vi "RealTimeStiffness.vi"() -> ()   [LabVIEW 2017]
uses:
  <vilib>/Utility/file.llb/Read Delimited Spreadsheet (DBL).vi
  <vilib>/Analysis/NI_AALBase.lvlib
panel:
  in  "Size":i32=500
  out "XY Graph":cluster{dbl[], dbl[]}[](graph)
  in  "Size":i32=60
  out "Histogram Graph":T1(graph)
  in  "stop":bool
  out "all rows":dbl[][](array[numeric])
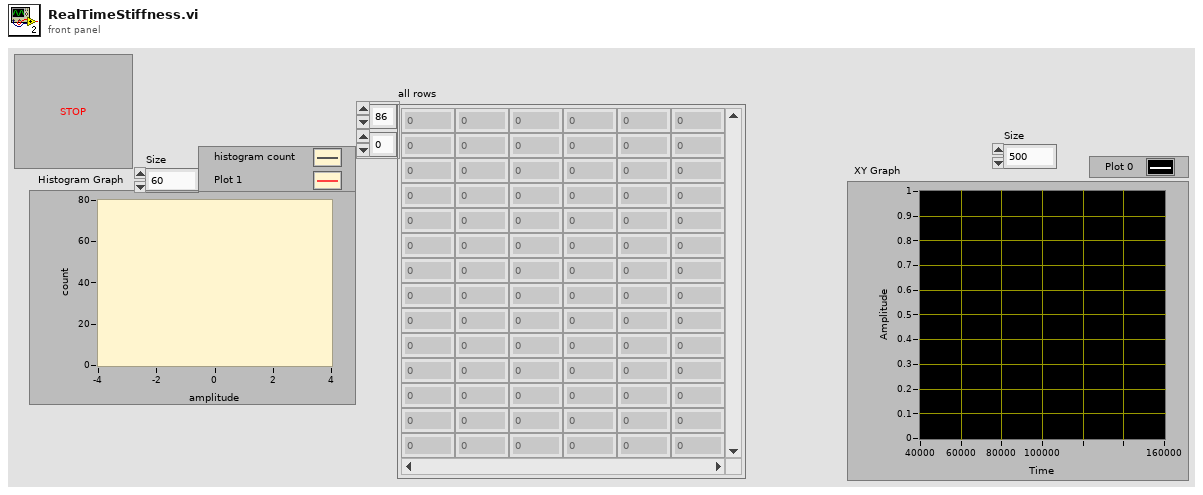
[diagram p1: front panel]
types:
  T1 = cluster{"X Values":dbl[], "Histogram: h(x)":i32[]}[]
  T2 = cluster{"X Values":dbl[], "Histogram: h(x)":i32[]}
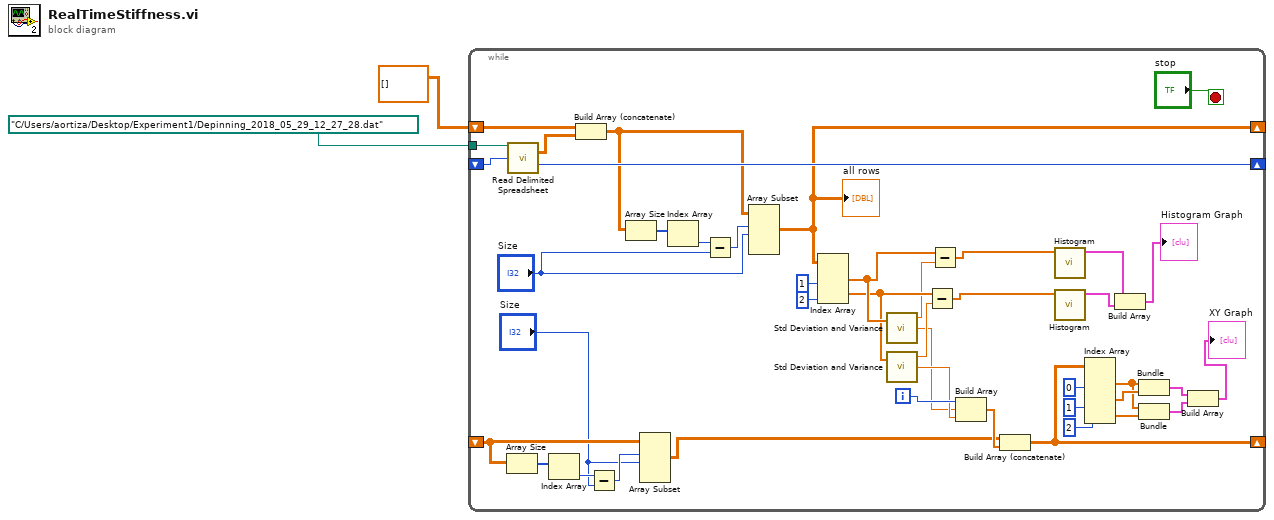
[diagram p0: block diagram]
diagram:
  n1 = while {
    tunnel: path "C:/Users/aortiza/Desktop/Experiment1/Depinning_2018_05_29_12_27_28.dat" ("file path (dialog if empty)") -> [w45]
    shift-right: [w35] -> _
    shift-left: dbl[][] [] -> [w38]
    shift-right: [w41] -> _
    shift-left: _ -> [w40]
    shift-right: [w16] -> _
    shift-left: _ -> [w20]
    i -> [w25]
    stop <- "stop" stop-if-true
    n2 = Array Size(array=w20) -> (size(s)=w22:i32[])
    n3 = call-poly <vilib>:"Read Delimited Spreadsheet.vi"("file path (dialog if empty)"=w45, "start of read offset (chars.:0)"=w40) -> ("all rows"=w37:dbl[][], "mark after read (chars.)"=w41:i32)  [unwired: 8 in, 4 out]
    n4 = Index Array(array=w22) -> (element=w19:i32)  [unwired: 1 in]
    n5 = Build Array (concatenate)(w38, w37) -> (w36:dbl[][])
    n6 = Subtract(x=w19, y="Size") -> (x-y=w18:i32)
    n7 = Array Size(array=w36) -> (size(s)=w44:i32[])
    n8 = Array Subset(array=w20, index (row)=w18, length (row)="Size") -> (w17:dbl[][])  [unwired: 2 in]
    n9 = Index Array(array=w44) -> (element=w43:i32)  [unwired: 1 in]
    n10 = Subtract(x=w43, y="Size") -> (x-y=w42:i32)
    n11 = Array Subset(array=w36, index (row)=w42, length (row)="Size") -> (w35:dbl[][])  [unwired: 2 in]
    "all rows" <- w35
    n12 = Index Array(array=w35, index (col) #1=1 ("disabled index (col)"), index (col) #2=2 ("index (col)")) -> (element #1=w28:dbl[], element #2=w27:dbl[])  [unwired: 2 in]
    n13 = call <vilib>:"Std Deviation and Variance.vi"("X"=w28) -> ("mean"=w24:dbl, "standard deviation"=w4:dbl)  [unwired: 1 in, 1 out]
    n14 = call <vilib>:"Std Deviation and Variance.vi"("X"=w27) -> ("mean"=w6:dbl, "standard deviation"=w5:dbl)  [unwired: 1 in, 1 out]
    n15 = Subtract(x=w27, y=w6) -> (x-y=w26:dbl[])
    n16 = Subtract(x=w28, y=w24) -> (x-y=w29:dbl[])
    n17 = Build Array(w25, w4, w5) -> (w23:dbl[])
    n18 = Build Array (concatenate)(w17, w23) -> (w16:dbl[][])
    n19 = call <vilib>:"Histogram.vi"("X"=w29) -> ("Histogram Graph"=w31:T2)  [unwired: 7 in, 3 out]
    n20 = call <vilib>:"Histogram.vi"("X"=w26) -> ("Histogram Graph"=w32:T2)  [unwired: 7 in, 3 out]
    n21 = Index Array(array=w16, index (col) #1=0 ("disabled index (col)"), index (col) #2=1 ("index (col)"), index (col) #3=2 ("index (col)")) -> (element #1=w11:dbl[], element #2=w12:dbl[], element #3=w10:dbl[])  [unwired: 3 in]
    n22 = Build Array(w31, w32) -> (→"Histogram Graph":T1)
    n23 = Bundle(w11, w12) -> (w9:cluster{dbl[], dbl[]})  [unwired: 1 in]
    n24 = Bundle(w11, w10) -> (w8:cluster{dbl[], dbl[]})  [unwired: 1 in]
    n25 = Build Array(w9, w8) -> (→"XY Graph":cluster{dbl[], dbl[]}[])
  }
